vi "Test1.vi"() -> ()   [LabVIEW 2013]
uses:
  <vilib>/Motion/MotorControl/_s/nism.digitalInputs.portA.ctl
  <vilib>/rvi/Emulation/niFpgaSctlEmulationGetInTimedLoop.vi
  <vilib>/rvi/Emulation/niFpgaEmulationReportErrorSimple.vi
  <vilib>/rvi/Emulation/niFpgaGetClockAttributes.vi
  Global FPGA 8-axis.vi
  <vilib>/Motion/MotorControl/_s/nism.interpretDIOControl.portA.single.2.vi
  <vilib>/Motion/MotorControl/_s/nism.generateDIOStatus.portA.single.vi
  <vilib>/rvi/Emulation/niFpgaCriticalErrorInLSC.vi
  <vilib>/Motion/MotorControl/NI_SoftMotion_MotorControlIP.lvlib
panel:
  in  "Axi1 1 DI":u8
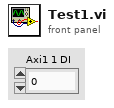
[diagram p1: front panel]
types:
  T1 = typedef "NI_SoftMotion_MotorControlIP.lvlib/nism.digitalInputs.portA.ctl" = cluster{"reverse limit":bool, "forward limit":bool, "home switch":bool, "digital input 0":bool, "digital input 1":bool, "digital input 2":bool, "digital input 3":bool}
  T2 = typedef "NI_SoftMotion_MotorControlIP.lvlib/nism.dio.portA.config.2.ctl" = cluster{"digital filter (us)":u16[], "safe state":enum16{"Low", "High", "No Change"}[]}
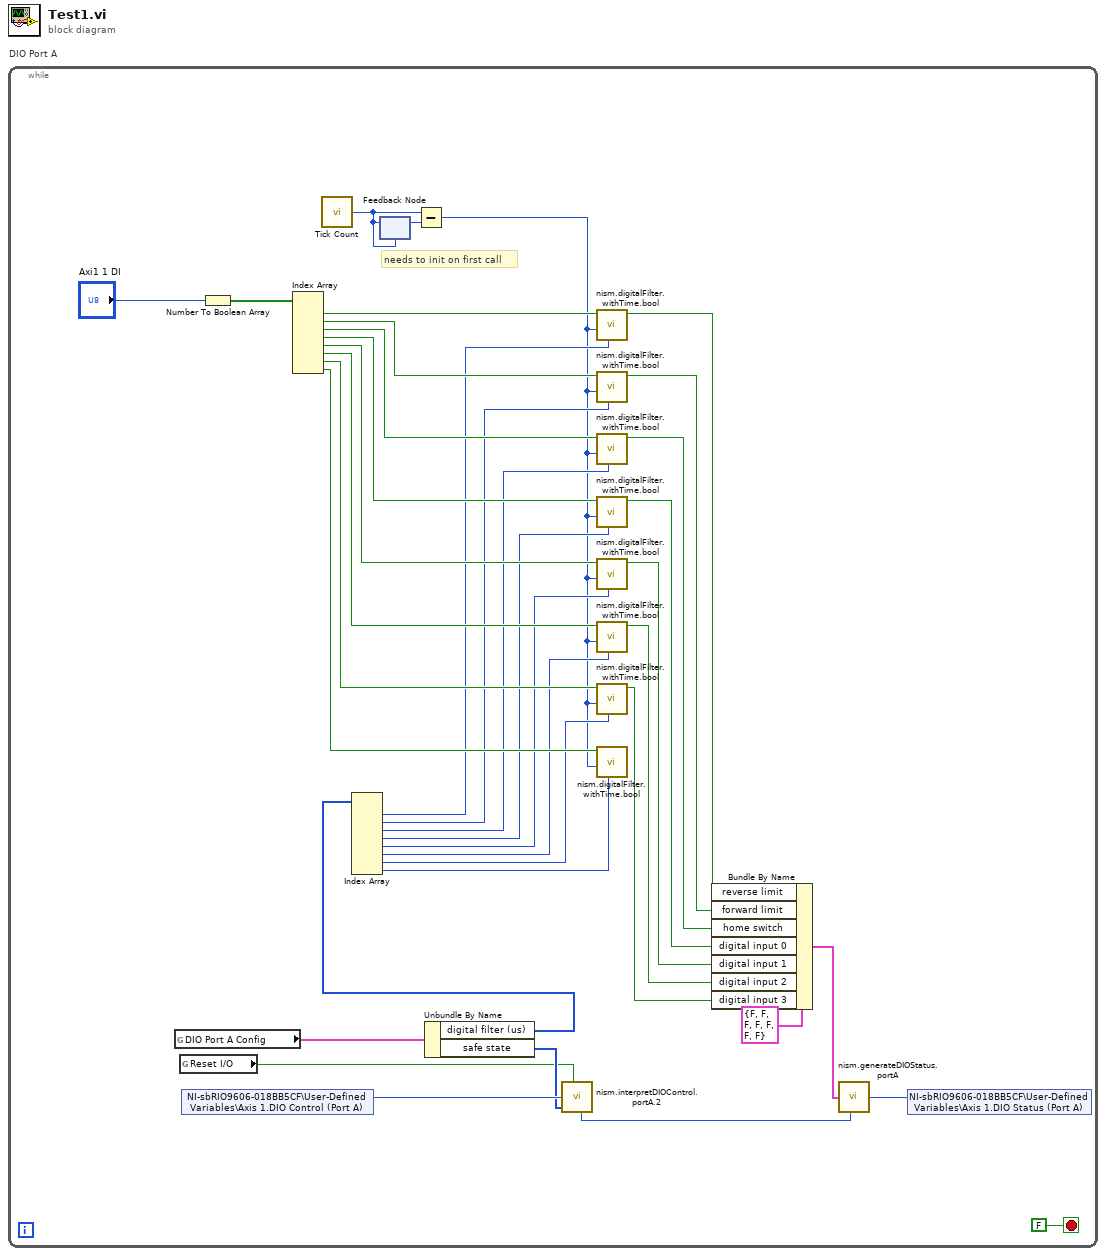
[diagram p0: block diagram]
diagram:
  n1 = while "DIO Port A" {
    stop <- FALSE stop-if-true
    # "needs to init on first call"
    n2 = global read "Global FPGA 8-axis.vi" "DIO Port A Config"() -> (w32:T2)
    n3 = global read "Global FPGA 8-axis.vi" "Reset I/O"() -> (w30:bool)
    n4 = shared-variable "NI-sbRIO9606-018BB5CF\\User-Defined Variables\\Axis 1.DIO Control (Port A)"() -> (w36:u32)  [unwired: 1 in, 1 out]
    n5 = Number To Boolean Array(number="Axi1 1 DI") -> (Boolean array=w28:bool[])
    n6 = Index Array(array=w28) -> (element #1=w27:bool, element #2=w20:bool, element #3=w21:bool, element #4=w22:bool, element #5=w23:bool, element #6=w24:bool, element #7=w25:bool, element #8=w26:bool)  [unwired: 8 in]
    n7 = call "Tick Count"() -> ("Tick Count(uSec)"=w10:u16)
    n8 = feedback #1(w10) -> (w11:u16)
    n9 = feedback-in #1(w10) -> ()
    n10 = Subtract(x=w10, y=w11) -> (x-y=w9:u16)
    n11 = Unbundle By Name(w32) -> ("digital filter (us)"=w8:u16[], "safe state"=w31:enum16{"Low", "High", "No Change"}[])
    n12 = Index Array(array=w8) -> (element #1=w12:u16, element #2=w13:u16, element #3=w14:u16, element #4=w15:u16, element #5=w16:u16, element #6=w17:u16, element #7=w18:u16, element #8=w19:u16)  [unwired: 8 in]
    n13 = call-poly <vilib>:"nism.interpretDIOControl.portA.2.vi"("reset"=w30, "dio control(port a)"=w36, "safe state"=w31) -> ("reset latches"=w38:u8)  [unwired: 5 in, 1 out]
    n14 = call <vilib>:"nism.digitalFilter.withTime.bool.vi"("filter value"=w12, "delta time"=w9, "input signal"=w27) -> ("output signal"=w7:bool)  [unwired: 8 in]
    n15 = call <vilib>:"nism.digitalFilter.withTime.bool.vi"("filter value"=w13, "delta time"=w9, "input signal"=w20) -> ("output signal"=w6:bool)  [unwired: 8 in]
    n16 = call <vilib>:"nism.digitalFilter.withTime.bool.vi"("filter value"=w14, "delta time"=w9, "input signal"=w21) -> ("output signal"=w5:bool)  [unwired: 8 in]
    n17 = call <vilib>:"nism.digitalFilter.withTime.bool.vi"("filter value"=w15, "delta time"=w9, "input signal"=w22) -> ("output signal"=w4:bool)  [unwired: 8 in]
    n18 = call <vilib>:"nism.digitalFilter.withTime.bool.vi"("filter value"=w16, "delta time"=w9, "input signal"=w23) -> ("output signal"=w3:bool)  [unwired: 8 in]
    n19 = call <vilib>:"nism.digitalFilter.withTime.bool.vi"("filter value"=w17, "delta time"=w9, "input signal"=w24) -> ("output signal"=w2:bool)  [unwired: 8 in]
    n20 = call <vilib>:"nism.digitalFilter.withTime.bool.vi"("filter value"=w18, "delta time"=w9, "input signal"=w25) -> ("output signal"=w1:bool)  [unwired: 8 in]
    n21 = call <vilib>:"nism.digitalFilter.withTime.bool.vi"("filter value"=w19, "delta time"=w9, "input signal"=w26) -> ()  [unwired: 8 in, 1 out]
    n22 = Bundle By Name(cluster=T1 {"reverse limit"=FALSE, "forward limit"=FALSE, "home switch"=FALSE, "digital input 0"=FALSE, "digital input 1"=FALSE, "digital input 2"=FALSE, "digital input 3"=FALSE} ("$(driveInterface.digitalInputs.shortName)"), "reverse limit"=w7, "forward limit"=w6, "home switch"=w5, "digital input 0"=w4, "digital input 1"=w3, "digital input 2"=w2, "digital input 3"=w1) -> (w34:T1)
    n23 = call-poly <vilib>:"nism.generateDIOStatus.portA.vi"("digital inputs"=w34, "reset latches"=w38) -> ("dio status(port a)"=w37:u32)  [unwired: 7 in]
    n24 = shared-variable "NI-sbRIO9606-018BB5CF\\User-Defined Variables\\Axis 1.DIO Status (Port A)"(w37) -> ()  [unwired: 1 in, 1 out]
  }
